vi "setupVersion_May13.vi"() -> (2 "Keithley 2100 out":bool, 3 "Keithley 6431":bool, 4 "J-KEM2":bool, 6 "Keithley 2421":bool, 8 "SRS QCM 2":bool, 10 "error IO":errorcluster, 12 "Arduino2":bool, 14 "Pressure control 2":bool, 15 "Save file path 2":path)   [LabVIEW 2014]
panel:
  in  "Instruments connected":T1
  in  "Save file path":path
  in  "OK":bool
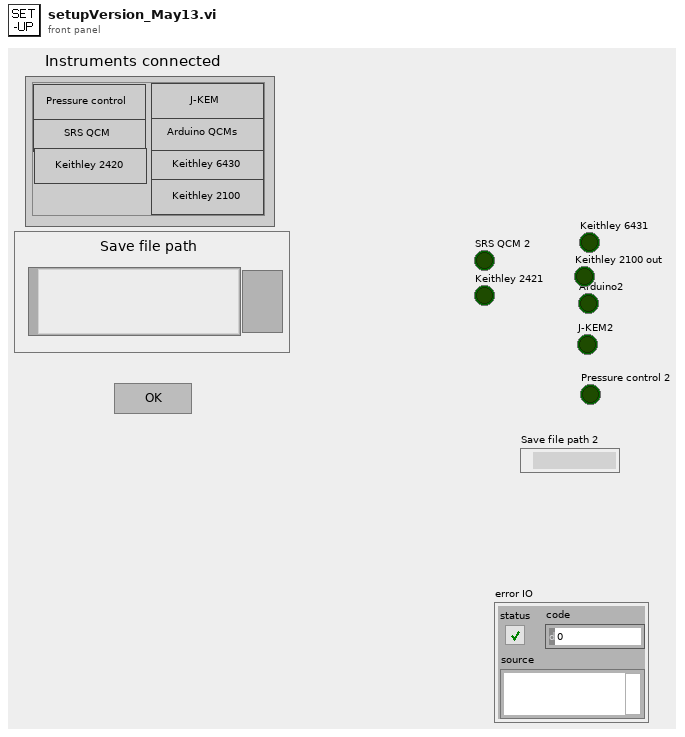
[diagram p1: front panel]
types:
  T1 = cluster{"SRS QCM":bool, "Keithley 2420":bool, "Keithley 6430":bool, "Keithley 2100":bool, "Arduino":bool, "J-KEM":bool, "Pressure control":bool}
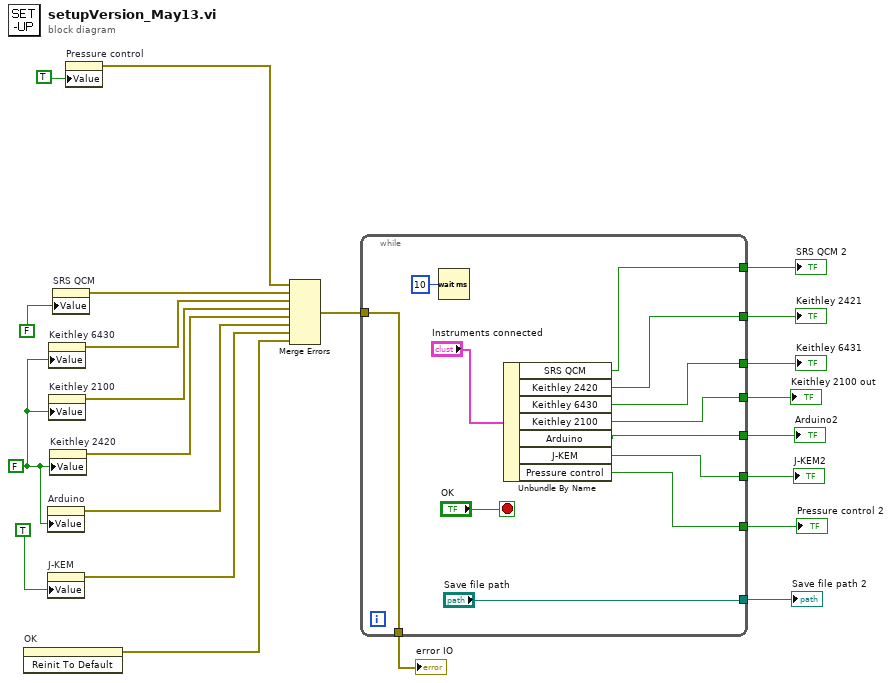
[diagram p0: block diagram]
diagram:
  w2 = FALSE ("Auto Stop")
  n1 = invoke on="OK" class="Bool" method="Reinit To Default"() -> (error out=w17:errorcluster)  [unwired: 3 in, 2 out]
  n2 = property on="Arduino" class="Bool (strict)"("Value"=w2) -> (error out=w12:errorcluster)  [unwired: 2 in, 1 out]
  n3 = property on="J-KEM" class="Bool (strict)"("Value"=TRUE ("Auto Stop")) -> (error out=w10:errorcluster)  [unwired: 2 in, 1 out]
  n4 = property on="Keithley 6430" class="Bool (strict)"("Value"=w2) -> (error out=w14:errorcluster)  [unwired: 2 in, 1 out]
  n5 = property on="Keithley 2100" class="Bool (strict)"("Value"=w2) -> (error out=w1:errorcluster)  [unwired: 2 in, 1 out]
  n6 = property on="Keithley 2420" class="Bool (strict)"("Value"=w2) -> (error out=w16:errorcluster)  [unwired: 2 in, 1 out]
  n7 = property on="SRS QCM" class="Bool (strict)"("Value"=FALSE ("Auto Stop")) -> (error out=w13:errorcluster)  [unwired: 2 in, 1 out]
  n8 = property on="Pressure control" class="Bool (strict)"("Value"=TRUE ("Auto Stop")) -> (error out=w4:errorcluster)  [unwired: 2 in, 1 out]
  n9 = Merge Errors(w4, w13, w14, w1, w16, w12, w10, w17) -> (w22:errorcluster)
  n10 = while {
    tunnel: w22 -> [w31]
    tunnel: [w29] -> w21
    tunnel: [w28] -> w20
    tunnel: [w27] -> w19
    tunnel: [w25] -> w18
    tunnel: [w24] -> w11
    tunnel: [w23] -> w8
    tunnel: ["Save file path"] -> w7
    tunnel: [w31] -> w5
    tunnel: [w26] -> w3
    stop <- "OK" stop-if-true
    n11 = Wait (ms)(milliseconds to wait=u32 10) -> ()  [unwired: 1 out]
    n12 = Unbundle By Name("Instruments connected") -> ("SRS QCM"=w29:bool, "Keithley 2420"=w28:bool, "Keithley 6430"=w27:bool, "Keithley 2100"=w26:bool, "Arduino"=w25:bool, "J-KEM"=w24:bool, "Pressure control"=w23:bool)
  }
  "SRS QCM 2" <- w21
  "Keithley 2421" <- w20
  "Keithley 6431" <- w19
  "Arduino2" <- w18
  "J-KEM2" <- w11
  "Pressure control 2" <- w8
  "Save file path 2" <- w7
  "error IO" <- w5
  "Keithley 2100 out" <- w3
